vi "Get RPM.vi"() -> (0 "Main RPM":dbl, 1 "Pre RPM":dbl)   [LabVIEW 2013]
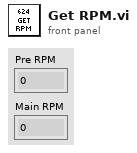
[diagram p1: front panel]
types:
  T1 = typedef "WPI_CounterDevRef.ctl" = cluster{"DevStatus":errorcluster, "CntIndex":T2}
  T2 = typedef "FPGA_CounterCtrSystemIndex.ctl" = enum8{"Ctr 0", "Ctr 1", "Ctr 2", "Ctr 3", "Ctr 4", "Ctr 5", "Ctr 6", "Ctr 7", "Invalid"}
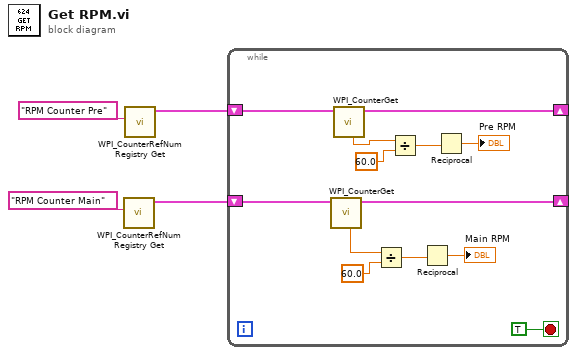
[diagram p0: block diagram]
diagram:
  n1 = call <vilib>:"WPI_CounterRefNum Registry Get.vi"("refnum name"="RPM Counter Main") -> ("CounterDevRef"=w2:T1)  [unwired: 9 in, 1 out]
  n2 = call <vilib>:"WPI_CounterRefNum Registry Get.vi"("refnum name"="RPM Counter Pre") -> ("CounterDevRef"=w1:T1)  [unwired: 9 in, 1 out]
  n3 = while {
    shift-right: [w7] -> _
    shift-left: w1 -> [w10]
    shift-right: [w8] -> _
    shift-left: w2 -> [w11]
    stop <- TRUE stop-if-true
    n4 = call <vilib>:"WPI_CounterGet.vi"("CounterDevRef in"=w11) -> ("CounterDevRef out"=w8:T1, "Period (sec)"=w12:dbl)  [unwired: 5 in, 4 out]
    n5 = call <vilib>:"WPI_CounterGet.vi"("CounterDevRef in"=w10) -> ("CounterDevRef out"=w7:T1, "Period (sec)"=w17:dbl)  [unwired: 5 in, 4 out]
    n6 = Divide(x=w12, y=60.0) -> (x/y=w14:dbl)
    n7 = Divide(x=w17, y=60.0) -> (x/y=w15:dbl)
    n8 = Reciprocal(x=w14) -> (1/x=→"Main RPM":dbl)
    n9 = Reciprocal(x=w15) -> (1/x=→"Pre RPM":dbl)
  }
